vi "rad_Configure Blacklists.vi"(8 "error in (no error)":errorcluster, 11 "AppImage Properties In":T1) -> (0 "error out":errorcluster, 2 "Canceled":bool, 3 "AppImage Properties Out":T1)   [LabVIEW 2014]
uses:
  TypeDefs/rad_Blacklist Object.ctl
  TypeDefs/rad_FPGA Flash Properties.ctl
  TypeDefs/rad_FPGA Properties.ctl
  TypeDefs/rad_Application Image Properties.ctl
panel:
  in  "Explain This":bool
  in  "Add":bool
  in  "Save":bool
  in  "Cancel":bool
  out "Blacklist Folders / Files":T4[](array[typedef])
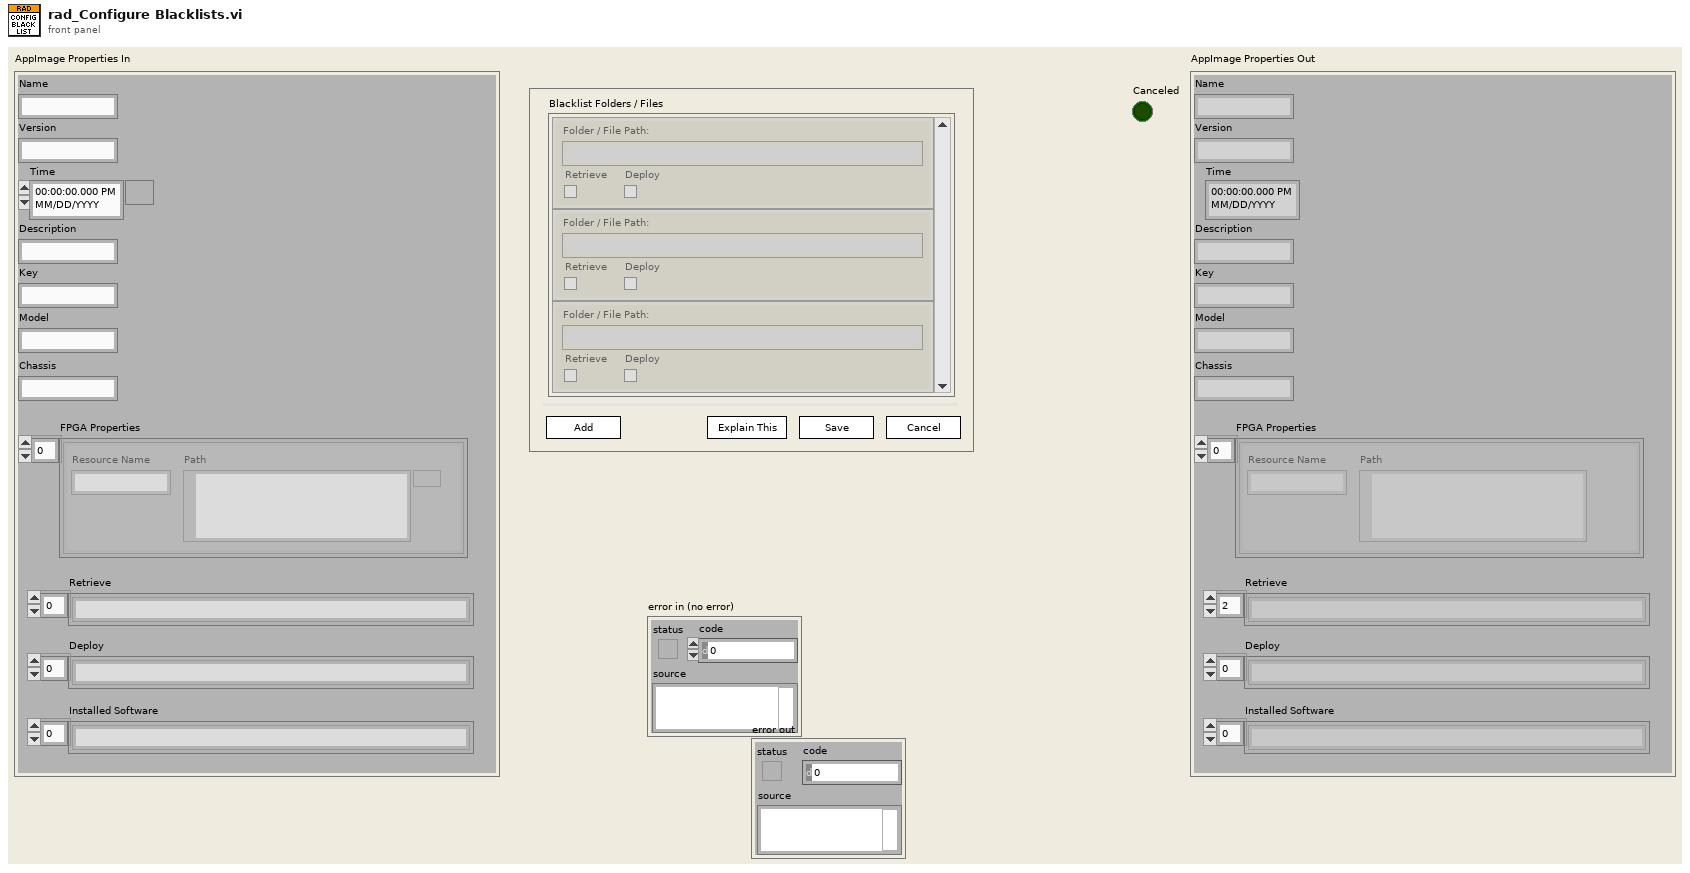
[diagram p1: front panel]
types:
  T1 = typedef "rad_Application Image Properties.ctl" = cluster{"Name":string, "Version":string, "Time":timestamp, "Description":string, "Key":string, "Chassis":string, "FPGA Properties":T2, "Model":string, "Retrieve":string[], "Deploy":string[], "Installed Software":string[]}
  T2 = typedef "rad_FPGA Properties.ctl" = T3[]
  T3 = typedef "rad_FPGA Flash Properties.ctl" = cluster{"Resource Name":string, "Path":path}
  T4 = typedef "rad_Blacklist Object.ctl" = cluster{"Folder / File Path:":string, "Retrieve":bool, "Deploy":bool}
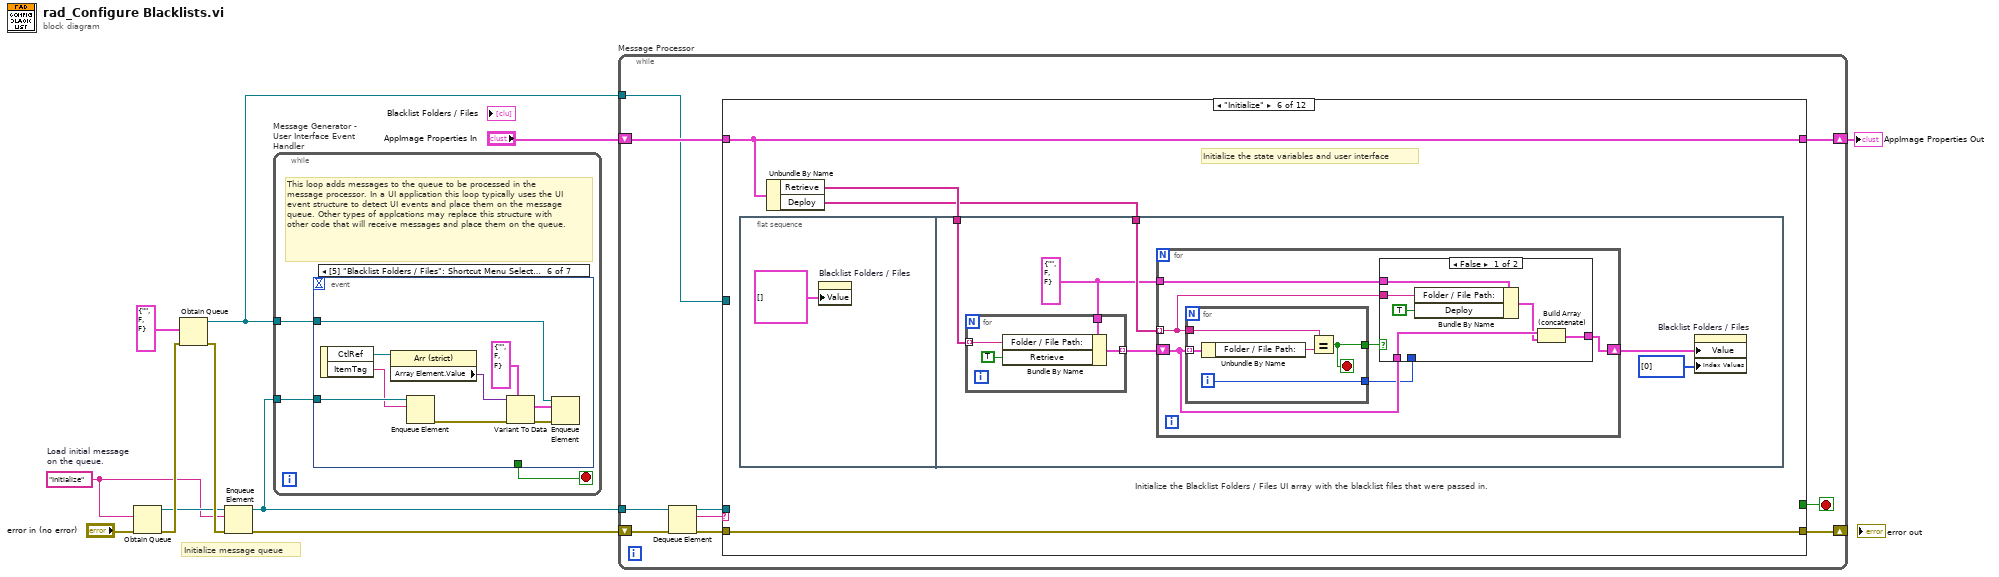
[diagram p0: block diagram]
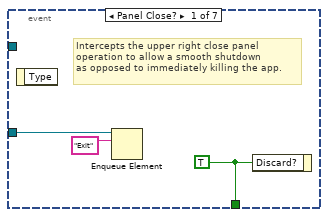
[diagram p2: hidden frame]
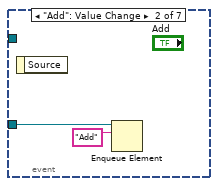
[diagram p3: hidden frame]
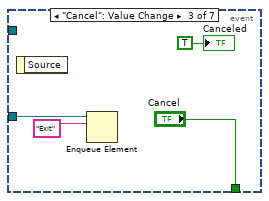
[diagram p4: hidden frame]
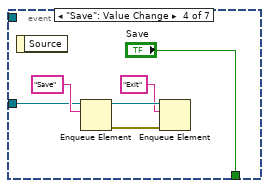
[diagram p5: hidden frame]
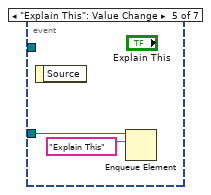
[diagram p6: hidden frame]
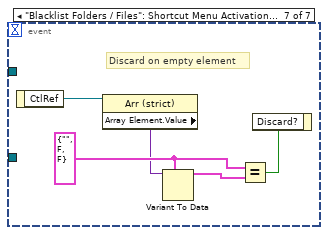
[diagram p7: hidden frame]
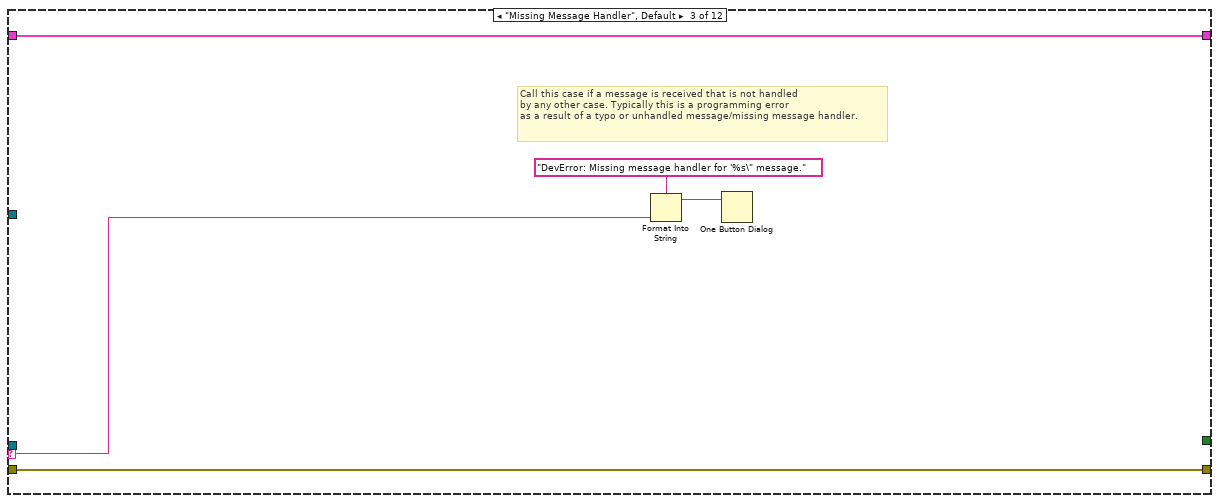
[diagram p10: hidden frame]
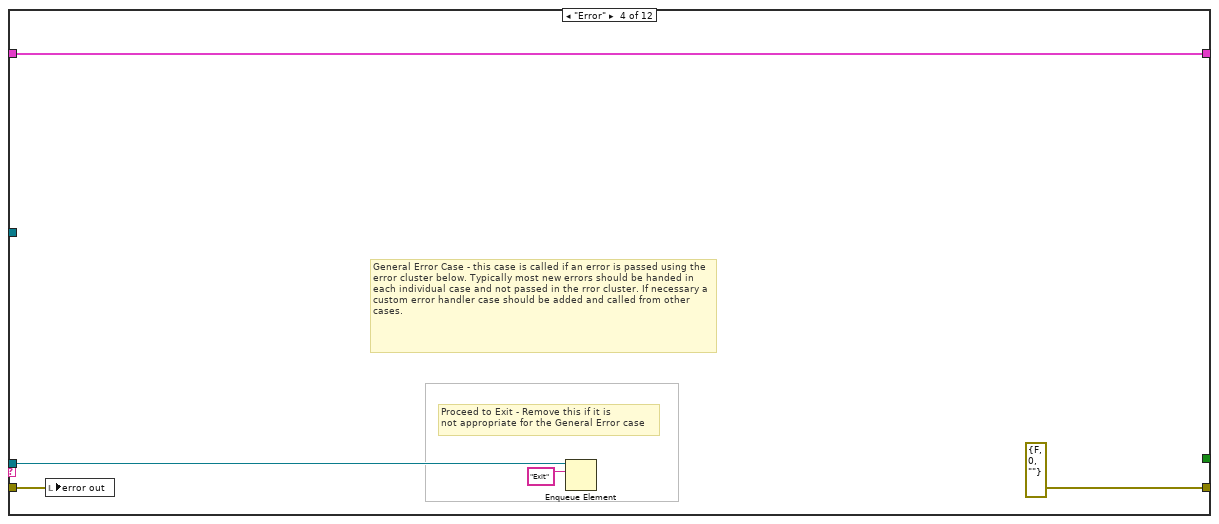
[diagram p11: hidden frame]
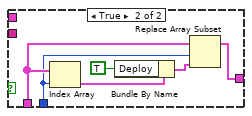
[diagram p13: hidden frame]
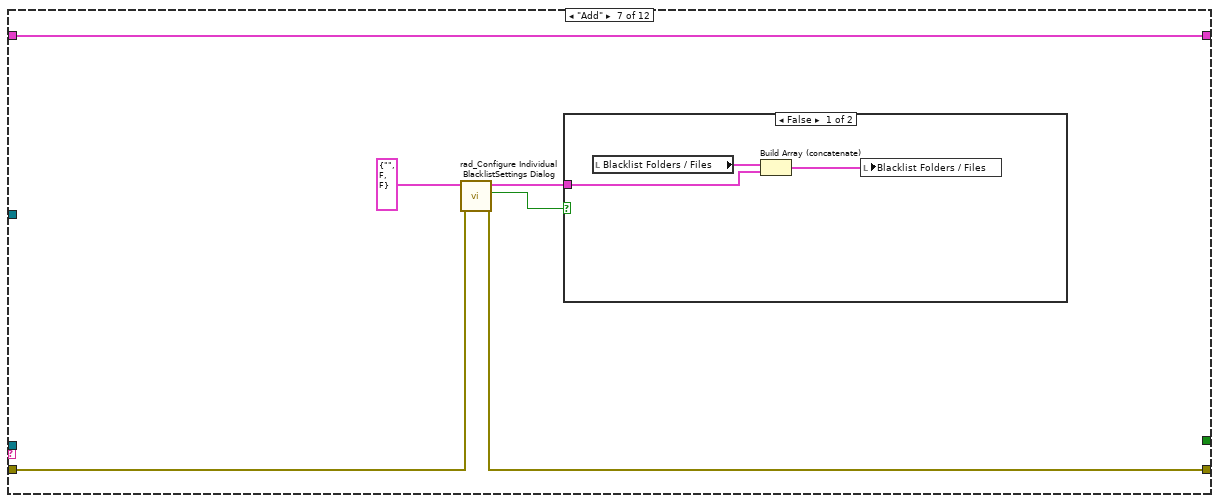
[diagram p14: hidden frame]
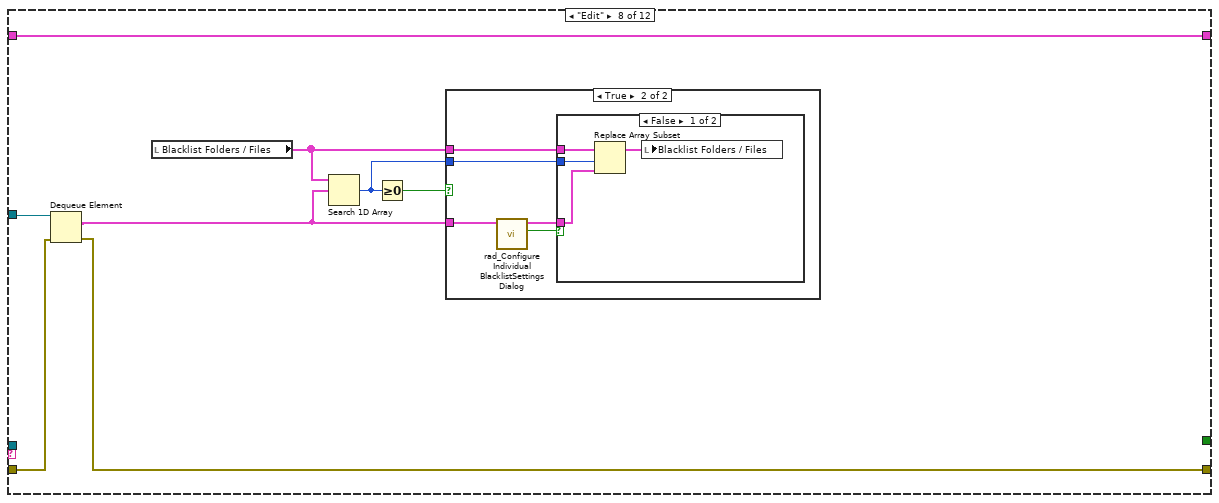
[diagram p16: hidden frame]
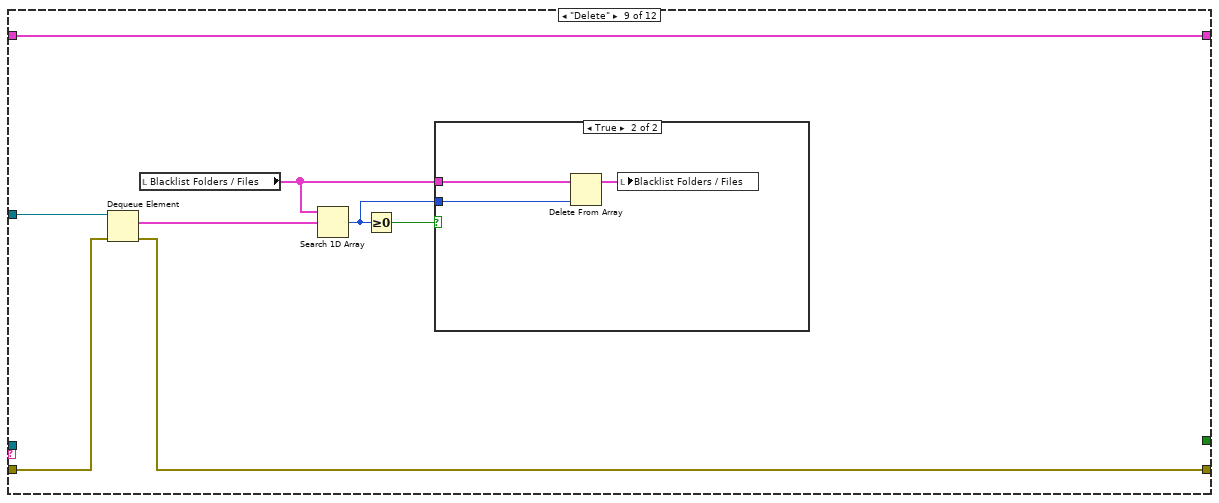
[diagram p19: hidden frame]
diagram:
  w2 = "Initialize"  # Load initial message on the queue.
  # "Initialize message queue"
  n1 = Obtain Queue(element data type=w2, error in (no error)="error in (no error)") -> (queue out=w3:refnum<queue>, error out=w5:errorcluster)  [unwired: 3 in, 1 out]
  n2 = Obtain Queue(element data type=T4 {"Folder / File Path:"="", "Retrieve"=FALSE, "Deploy"=FALSE} ("blacklistObject"), error in (no error)=w5) -> (queue out=w1:refnum<queue>, error out=w4:errorcluster)  [unwired: 3 in, 1 out]
  n3 = Enqueue Element(queue=w3, element=w2, error in (no error)=w4) -> (queue out=w11:refnum<queue>, error out=w10:errorcluster)  [unwired: 1 in, 1 out]
  n4 = while "Message Generator - User Interface Event Handler" {
    tunnel: w11 -> [w13]
    tunnel: w1 -> [w12]
    stop <- w14 stop-if-true
    # "This loop adds messages to the queue to be processed in the message processor. In a UI application this loop typically uses the UI event structure to detect UI events and place them on the message queue. Other types of applcations may replace this structure with other code that will receive messages and place them on the queue."
    n5 = event shown="[5] \"Blacklist Folders / Files\": Shortcut Menu Selection (User)" {
      selector: _ -> [_ _ _ _ _ _ _]
      dyn-events: _ -> [_ _ _ _ _ _ _]
      timeout: _ -> [_ _ _ _ _ _ _]
      tunnel: [w17 _ "Cancel" "Save" _ _ _] -> w14
      tunnel: w13 -> [w15 w18 w22 w28 w30 w39 _]
      tunnel: w12 -> [_ _ _ _ _ w34 _]
      event Panel Close? {
        w17 = TRUE ("Discard?")
        # "Intercepts the upper right close panel\noperation to allow a smooth shutdown\nas opposed to immediately killing the app."
        n6 = event-data() -> ()  [unwired: 2 out]
        n7 = Enqueue Element(queue=w15, element="Exit") -> ()  [unwired: 2 in, 3 out]
        n8 = event-data("Discard?"=w17) -> ()  [unwired: 1 in, 1 out]
      }
      event "Add": Value Change {
        n9 = event-data() -> ()  [unwired: 2 out]
        n10 = Enqueue Element(queue=w18, element="Add") -> ()  [unwired: 2 in, 3 out]
      }
      event "Cancel": Value Change {
        n11 = event-data() -> ()  [unwired: 2 out]
        n12 = Enqueue Element(queue=w22, element="Exit") -> ()  [unwired: 2 in, 3 out]
        "Canceled" <- TRUE
      }
      event "Save": Value Change {
        n13 = event-data() -> ()  [unwired: 2 out]
        n14 = Enqueue Element(queue=w28, element="Save") -> (queue out=w27:refnum<queue>, error out=w24:errorcluster)  [unwired: 2 in, 1 out]
        n15 = Enqueue Element(queue=w27, element="Exit" ("Message Name"), error in (no error)=w24) -> ()  [unwired: 1 in, 3 out]
      }
      event "Explain This": Value Change {
        n16 = event-data() -> ()  [unwired: 2 out]
        n17 = Enqueue Element(queue=w30, element="Explain This" ("Message Name")) -> ()  [unwired: 2 in, 3 out]
      }
      event "Blacklist Folders / Files": Shortcut Menu Selection (User) {
        n18 = event-data() -> ("CtlRef"=w40:refnum<vi>, "ItemTag"=w38:string)  [unwired: 1 out]
        n19 = property class="Arr (strict)"(reference=w40) -> ("Array Element.Value"=w36:variant)  [unwired: 1 in, 2 out]
        n20 = Enqueue Element(queue=w39, element=w38) -> (error out=w33:errorcluster)  [unwired: 2 in, 2 out]
        n21 = Variant To Data(error in=w33, type=T4 {"Folder / File Path:"="", "Retrieve"=FALSE, "Deploy"=FALSE} ("blacklistObject"), Variant=w36) -> (data=w35:T4, error out=w32:errorcluster)
        n22 = Enqueue Element(queue=w34, element=w35, error in (no error)=w32) -> ()  [unwired: 1 in, 3 out]
      }
      event "Blacklist Folders / Files": Shortcut Menu Activation? {
        w44 = T4 {"Folder / File Path:"="", "Retrieve"=FALSE, "Deploy"=FALSE} ("blacklistObject")
        # "Discard on empty element"
        n23 = event-data() -> ("CtlRef"=w45:refnum<vi>)  [unwired: 1 out]
        n24 = property class="Arr (strict)"(reference=w45) -> ("Array Element.Value"=w42:variant)  [unwired: 1 in, 2 out]
        n25 = Variant To Data(type=w44, Variant=w42) -> (data=w43:T4)  [unwired: 1 in, 1 out]
        n26 = Equal?(x=w44, y=w43) -> (x = y?=w41:bool)
        n27 = event-data("Discard?"=w41) -> ()  [unwired: 1 in, 1 out]
      }
    }
  }
  n28 = while "Message Processor" {
    shift-left: w10 -> [w50]
    shift-right: [w53] -> _
    tunnel: w11 -> [w51]
    shift-left: "AppImage Properties In" -> [w55]
    shift-right: [w54] -> w9
    tunnel: w1 -> [w46]
    stop <- w47 stop-if-true
    n29 = Dequeue Element(queue=w51, error in (no error)=w50) -> (queue out=w52:refnum<queue>, element=w48:string, error out=w49:errorcluster)  [unwired: 1 in, 1 out]
    n30 = case shown="\"Initialize\"" w48 {
      selector: w48 -> [_ _ w62 _ _ _ _ _ _ _ _ _]
      tunnel: [w57 w59 w64 w69 w71 w74 w115 w126 w143 w150 w171 w179] -> w54
      tunnel: w55 -> [w57 w59 w64 w69 w71 w74 w115 w126 w143 w151 w171 w179]
      tunnel: w52 -> [_ _ _ w67 _ _ _ _ _ _ _ w177]
      tunnel: w49 -> [w56 w58 w63 w65 w70 w75 w114 w121 w137 w149 w172 w178]
      tunnel: [w56 w58 w63 errorcluster {"status"=FALSE, "code"=0, "source"=""} ("error out") w70 w75 w113 w120 w136 w149 w172 w173] -> w53
      tunnel: w46 -> [_ _ _ _ _ _ _ w122 w138 _ _ w175]
      tunnel: [_ _ _ _ _ _ _ _ _ _ _ TRUE] -> w47
      frame "---------- Framework Operations ----------" {
        # "Dummy case to add a seperator in the Case Structure menu"
      }
      frame "", "Idle" {
        # "Idle Case - this case is called after a Timeout on the Get Next Message from Queue VI, if no new messages are present on the queue. This case can be used for housekeeping tasks such as updating the UI."
      }
      frame "Missing Message Handler", Default {
        # "Call this case if a message is received that is not handled \nby any other case. Typically this is a programming error\nas a result of a typo or unhandled message/missing message handler."
        n31 = Format Into String(format string="DevError: Missing message handler for '%s\" message." ("message"), w62) -> (resulting string=w60:string)  [unwired: 2 in, 1 out]
        n32 = One Button Dialog(message=w60) -> ()  [unwired: 2 out]
      }
      frame "Error" {
        # "Proceed to Exit - Remove this if it is\nnot appropriate for the General Error case"
        # "General Error Case - this case is called if an error is passed using the error cluster below. Typically most new errors should be handed in each individual case and not passed in the rror cluster. If necessary a custom error handler case should be added and called from other cases."
        n33 = local write "error out"(w65) -> ()
        n34 = Enqueue Element(queue=w67, element="Exit") -> ()  [unwired: 2 in, 3 out]
      }
      frame "---------- Generic Operations ----------" {
        # "Dummy case to add a seperator in the Case Structure menu"
      }
      frame "Initialize" {
        # "Initialize the Blacklist Folders / Files UI array with the blacklist files that were passed in."
        # "Initialize the state variables and user interface"
        n35 = flat-sequence {
          tunnel: w73 -> [w82]
          tunnel: w72 -> [w81]
          frame #0 {
            n36 = property on="Blacklist Folders / Files" class="Arr (strict)"("Value"=T4[] [] ("Blacklist Folders / Files")) -> ()  [unwired: 2 in, 2 out]
          }
          frame #1 {
            w77 = T4 {"Folder / File Path:"="", "Retrieve"=FALSE, "Deploy"=FALSE} ("blacklistObject")
            n37 = for {
              tunnel: w82 -> [w106] mode=indexing
              tunnel: w77 -> [w109]
              tunnel: [w107] -> w80 mode=indexing
              n38 = Bundle By Name(cluster=w109, "Folder / File Path:"=w106, "Retrieve"=TRUE) -> (w107:T4)
            }
            n39 = for {
              tunnel: w81 -> [w88] mode=indexing
              tunnel: w77 -> [w87]
              shift-right: [w84] -> w78
              shift-left: w80 -> [w85]
              n40 = for {
                tunnel: w85 -> [w105] mode=indexing
                tunnel: w88 -> [w103]
                tunnel: [w102] -> w86
                tunnel: [w101] -> w83
                i -> [w101]
                stop <- w102 stop-if-true
                n41 = Unbundle By Name(w105) -> ("Folder / File Path:"=w104:string)
                n42 = Equal?(x=w103, y=w104) -> (x = y?=w102:bool)
              }
              n43 = case shown="False" w86 {
                tunnel: w88 -> [w94 _]
                tunnel: w87 -> [w93 _]
                tunnel: w85 -> [w91 w98]
                tunnel: [w89 w95] -> w84
                tunnel: w83 -> [_ w97]
                frame False {
                  n44 = Bundle By Name(cluster=w93, "Folder / File Path:"=w94, "Deploy"=TRUE) -> (w90:T4)
                  n45 = Build Array (concatenate)(w91, w90) -> (w89:T4[])
                }
                frame True {
                  n46 = Index Array(array=w98, index=w97) -> (element=w100:T4)
                  n47 = Bundle By Name(cluster=w100, "Deploy"=TRUE) -> (w96:T4)
                  n48 = Replace Array Subset(array=w98, new element=w96, index=w97) -> (w95:T4[])
                }
              }
            }
            n49 = property on="Blacklist Folders / Files" class="Arr (strict)"("Value"=w78, "Index Values"=u32[] [0]) -> ()  [unwired: 2 in, 2 out]
          }
        }
        n50 = Unbundle By Name(w74) -> ("Retrieve"=w73:string[], "Deploy"=w72:string[])
      }
      frame "Add" {
        n51 = call "rad_Configure Individual BlacklistSettings Dialog.vi"("error in (no error)"=w114, "blacklistObject In"=T4 {"Folder / File Path:"="", "Retrieve"=FALSE, "Deploy"=FALSE}) -> ("error out"=w113:errorcluster, "Canceled"=w112:bool, "blacklistObject Out"=w111:T4)  [unwired: 7 in]
        n52 = case shown="False" w112 {
          tunnel: w111 -> [w117 _]
          frame False {
            n53 = local read "Blacklist Folders / Files"() -> (w118:T4[])
            n54 = Build Array (concatenate)(w118, w117) -> (w116:T4[])
            n55 = local write "Blacklist Folders / Files"(w116) -> ()
          }
          frame True {
          }
        }
      }
      frame "Edit" {
        n56 = Dequeue Element(queue=w122, error in (no error)=w121) -> (element=w119:T4, error out=w120:errorcluster)  [unwired: 1 in, 2 out]
        n57 = local read "Blacklist Folders / Files"() -> (w124:T4[])
        n58 = Search 1D Array(1D array=w124, element=w119) -> (index of element=w123:i32)  [unwired: 1 in]
        n59 = Greater Or Equal To 0?(x=w123) -> (x >= 0?=w125:bool)
        n60 = case shown="True" w125 {
          tunnel: w119 -> [_ w131]
          tunnel: w124 -> [_ w128]
          tunnel: w123 -> [_ w127]
          frame False {
          }
          frame True {
            n61 = call "rad_Configure Individual BlacklistSettings Dialog.vi"("blacklistObject In"=w131) -> ("Canceled"=w130:bool, "blacklistObject Out"=w129:T4)  [unwired: 8 in, 1 out]
            n62 = case shown="False" w130 {
              tunnel: w129 -> [w133 _]
              tunnel: w128 -> [w135 _]
              tunnel: w127 -> [w134 _]
              frame False {
                n63 = Replace Array Subset(array=w135, new element=w133, index=w134) -> (w132:T4[])
                n64 = local write "Blacklist Folders / Files"(w132) -> ()
              }
              frame True {
              }
            }
          }
        }
      }
      frame "Delete" {
        n65 = Dequeue Element(queue=w138, error in (no error)=w137) -> (element=w140:T4, error out=w136:errorcluster)  [unwired: 1 in, 2 out]
        n66 = local read "Blacklist Folders / Files"() -> (w139:T4[])
        n67 = Search 1D Array(1D array=w139, element=w140) -> (index of element=w141:i32)  [unwired: 1 in]
        n68 = Greater Or Equal To 0?(x=w141) -> (x >= 0?=w142:bool)
        n69 = case shown="True" w142 {
          tunnel: w139 -> [_ w146]
          tunnel: w141 -> [_ w144]
          frame False {
          }
          frame True {
            n70 = Delete From Array(array=w146, index=w144) -> (array with subset deleted=w145:T4[])  [unwired: 1 in, 1 out]
            n71 = local write "Blacklist Folders / Files"(w145) -> ()
          }
        }
      }
      frame "Save" {
        n72 = property on="Blacklist Folders / Files" class="Arr (strict)"() -> ("Value"=w152:T4[])  [unwired: 2 in, 2 out]
        n73 = for {
          tunnel: w152 -> [w162] mode=indexing
          shift-right: [w158] -> w148
          shift-left: string[] [] -> [w155]
          shift-right: [w157] -> w147
          shift-left: string[] [] -> [w156]
          n74 = Unbundle By Name(w162) -> ("Folder / File Path:"=w159:string, "Retrieve"=w161:bool, "Deploy"=w160:bool)
          n75 = case shown="True" w161 {
            tunnel: w155 -> [w167 w170]
            tunnel: w159 -> [_ w168]
            tunnel: [w167 w169] -> w158
            frame False {
            }
            frame True {
              n76 = Build Array (concatenate)(w170, w168) -> (w169:string[])
            }
          }
          n77 = case shown="True" w160 {
            tunnel: w156 -> [w163 w166]
            tunnel: w159 -> [_ w165]
            tunnel: [w163 w164] -> w157
            frame False {
            }
            frame True {
              n78 = Build Array (concatenate)(w166, w165) -> (w164:string[])
            }
          }
        }
        n79 = Bundle By Name(cluster=w151, "Retrieve"=w148, "Deploy"=w147) -> (w150:T1)
      }
      frame "Explain This" {
        n80 = call "rad_Blacklist Help.vi"() -> ()  [unwired: 12 in]
      }
      frame "Exit" {
        # "Stop the VI\n>> Perform any cleanup tasks in this message case.\n>> Clear display before closing."
        n81 = Release Queue(queue=w177, error in (no error)=w178) -> (error out=w174:errorcluster)  [unwired: 1 in, 2 out]
        n82 = Release Queue(queue=w175, error in (no error)=w174) -> (error out=w173:errorcluster)  [unwired: 1 in, 2 out]
      }
    }
  }
  "AppImage Properties Out" <- w9
